vi "GetCurrent__slk_tc.vi"(0 "tree control in":refnum<class "TreeControl.lvclass">, 11 "error in (no error)":errorcluster, 12 "column # (0)":i32) -> (4 "tree control out":refnum<class "TreeControl.lvclass">, 6 "current tag":string, 10 "current text":string, 15 "error out":errorcluster)   [LabVIEW 2020, in "TreeControl.lvclass"]
doc: "Retrieves the currently selected item in the tree. Requires that the tree selection property be set to no more than 1 element."
uses:
  Library/TreeControl.lvclass
  Library/TreeControl.lvclass/TreeControl.ctl
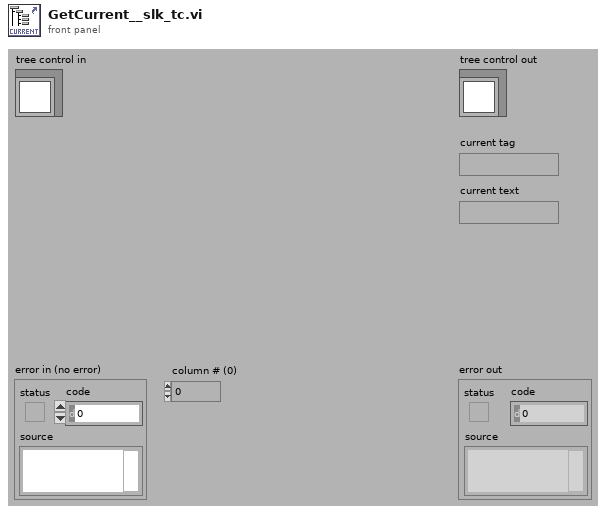
[diagram p1: front panel]
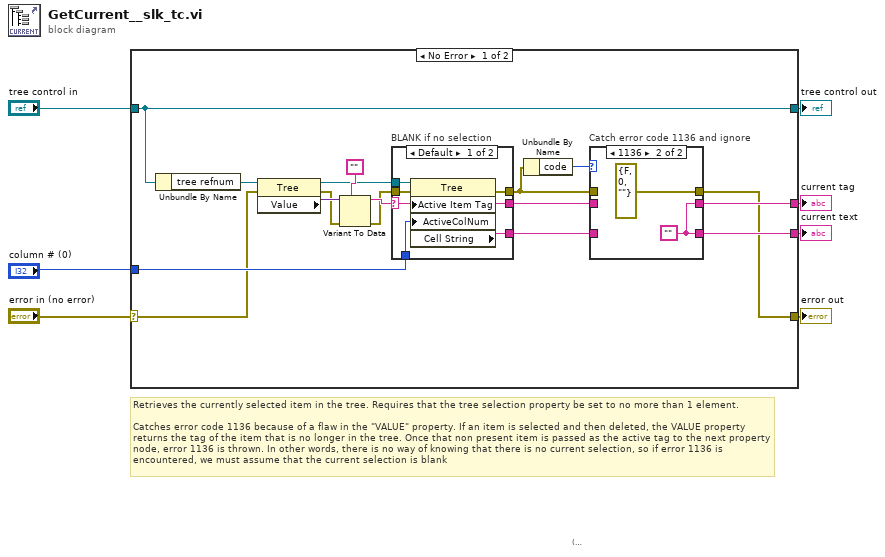
[diagram p0: block diagram]
diagram:
  # "(c)"
  # "Retrieves the currently selected item in the tree. Requires that the tree selection property be set to no more than 1 element. \n\nCatches error code 1136 because of a flaw in the \"VALUE\" property. If an item is selected and then deleted, the VALUE property returns the tag of the item that is no longer in the tree. Once that non present item is passed as the active tag to the next property node, error 1136 is thrown. In other words, there is no way of knowing that there is no current selection, so if error 1136 is encountered, we must assume that the current selection is blank"
  n1 = case shown="No Error" "error in (no error)" {
    selector: "error in (no error)" -> [w9 w39]
    tunnel: [w8 w39] -> w6
    tunnel: [w24 w38] -> w4
    tunnel: "tree control in" -> [w24 w38]
    tunnel: "column # (0)" -> [w16 _]
    tunnel: [w13 _] -> w1
    tunnel: [w11 _] -> w2
    frame No Error {
      n2 = Unbundle By Name(w24) -> ("tree refnum"=w23:refnum<vi>)
      n3 = property class="Tree"(reference=w23, error in=w9) -> (reference out=w19:refnum<vi>, error out=w18:errorcluster, "Value"=w22:variant)
      n4 = Variant To Data(error in=w18, type="", Variant=w22) -> (data=w20:string, error out=w17:errorcluster)
      n5 = case "BLANK if no selection" shown="Default" w20 {
        selector: w20 -> [w30 w36]
        tunnel: w19 -> [w35 _]
        tunnel: w17 -> [w34 w37]
        tunnel: w16 -> [w33 _]
        tunnel: [w32 w37] -> w10
        tunnel: [w31 w36] -> w14
        tunnel: [w30 w36] -> w12
        frame Default {
          n6 = property class="Tree"(reference=w35, error in=w34, "Active Item Tag"=w30, "ActiveColNum"=w33) -> (error out=w32:errorcluster, "Cell String"=w31:string)  [unwired: 1 out]
        }
        frame "" {
        }
      }
      n7 = Unbundle By Name(w10) -> ("code"=w15:i32)
      n8 = case "Catch error code 1136 and ignore" shown="1136" w15 {
        tunnel: w14 -> [w27 _]
        tunnel: [w27 w28] -> w13
        tunnel: [w26 w28] -> w11
        tunnel: w12 -> [w26 _]
        tunnel: w10 -> [w25 _]
        tunnel: [w25 errorcluster {"status"=FALSE, "code"=0, "source"=""} ("error out")] -> w8
        frame Default {
        }
        frame 1136 {
          w28 = ""
        }
      }
    }
    frame Error {
    }
  }
  "error out" <- w6
  "tree control out" <- w4
  "current tag" <- w2
  "current text" <- w1
